vi "DAQ_DO_Table.vi"(8 "error in":errorcluster caption="entrée d'erreur", 10 "Readout time (s)":dbl=0.1, 11 "Exposure time (s)":dbl=0.1) -> (0 "error out":errorcluster caption="sortie d'erreur", 2 "Dimension":u32)   [LabVIEW 2025]
uses:
  Controls/TypeDef_FGV.ctl
  FGV/FGV_DO_Table.vi
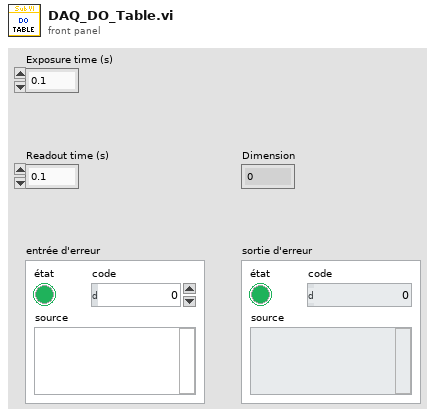
[diagram p1: front panel]
types:
  T1 = typedef "TypeDef_FGV.ctl" = enum16{"Initialize", "Write", "Read"}
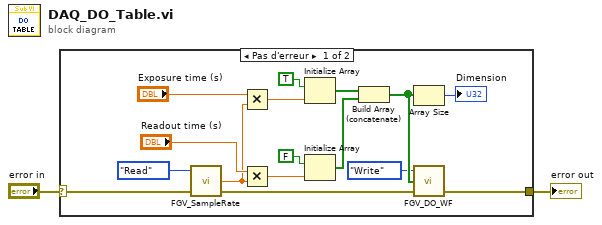
[diagram p0: block diagram]
diagram:
  n1 = case shown="Pas d'erreur" "error in" {
    selector: "error in" -> [w17 w19]
    tunnel: [w4 w19] -> w1
    frame No Error {
      n2 = call "FGV_SampleRate.vi"("error in"=w17, "Action"=TypeDef_FGV."Read") -> ("error out"=w6:errorcluster, "CO task"=w12:dbl)  [unwired: 2 in]
      n3 = Multiply(x="Exposure time (s)", y=w12) -> (x*y=w18:dbl)
      n4 = Multiply(x="Readout time (s)", y=w12) -> (x*y=w11:dbl)
      n5 = Initialize Array(TRUE, w18) -> (w10:bool[])
      n6 = Initialize Array(FALSE, w11) -> (w9:bool[])
      n7 = Build Array (concatenate)(w10, w9) -> (w5:bool[])
      n8 = Array Size(array=w5) -> (size(s)=→"Dimension":i32)
      n9 = call "FGV_DO_WF.vi"("error in"=w6, "DO table"=w5, "Action"=TypeDef_FGV."Write") -> ("error out"=w4:errorcluster)  [unwired: 1 in, 1 out]
    }
    frame Error {
    }
  }
  "error out" <- w1
